vi "Weighted Array Mean & SDV.vi"(4 "Reject NaN, +/-Inf (T)":bool=TRUE, 6 "Reject Negative Weights (F)":bool, 8 "Error In":errorcluster, 9 "Weight Array":dbl[](array[numeric]), 11 "Array":dbl[](array[numeric])) -> (0 "Error Out":errorcluster, 1 "SDV (weighted)":dbl, 2 "SDV (classic)":dbl, 3 "Average Value (weighted)":dbl, 5 "Average Value (classic)":dbl, 7 "Effective # Elements":i32)   [LabVIEW 2021, in "Math.lvlib"]
doc: "Compute a weighted average of the input <B>Array</B> A using the provided <B>Weight Array</B> w:\n\n<A> = (Sum(w_i A_i)_{i = 1....N})/(Sum(w_i)_{i = 1....N})\n\nwhere {A_i}_{i = 1....N} is the input <B>Array</B> and {w_i}_{i = 1....N} is the <B>Weight Array</B>.\n\nIf <B>Reject Negative Weights</B> is true, only the term with w_i >= 0 are retained in both sums.\n\nIf the two arrays have different sizes, the unweighted mean of <B>Array</B> is returned.\n\nTo reject NaN values in the calculation, use the <B>Reject NaN</B> flag."
uses:
  <userlib>/_OpenG.lib/array/array.llb/Filter 1D Array (DBL)__ogtk.vi
  <userlib>/_OpenG.lib/array/array.llb/Delete Elements from 1D Array (DBL)__ogtk.vi
  Math.lvlib
  <vilib>/Analysis/NI_AALBase.lvlib
  <userlib>/_OpenG.lib/array/array.llb/openg_array.lvlib
panel:
  # "see the AlliGator License on the block diagram (Ctrl+E or Window:Show Block Diagram)"
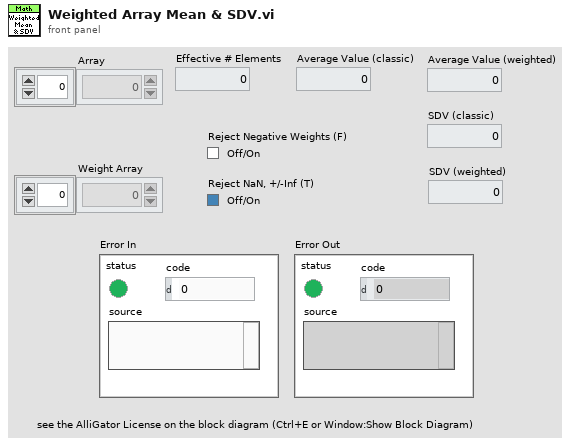
[diagram p1: front panel]
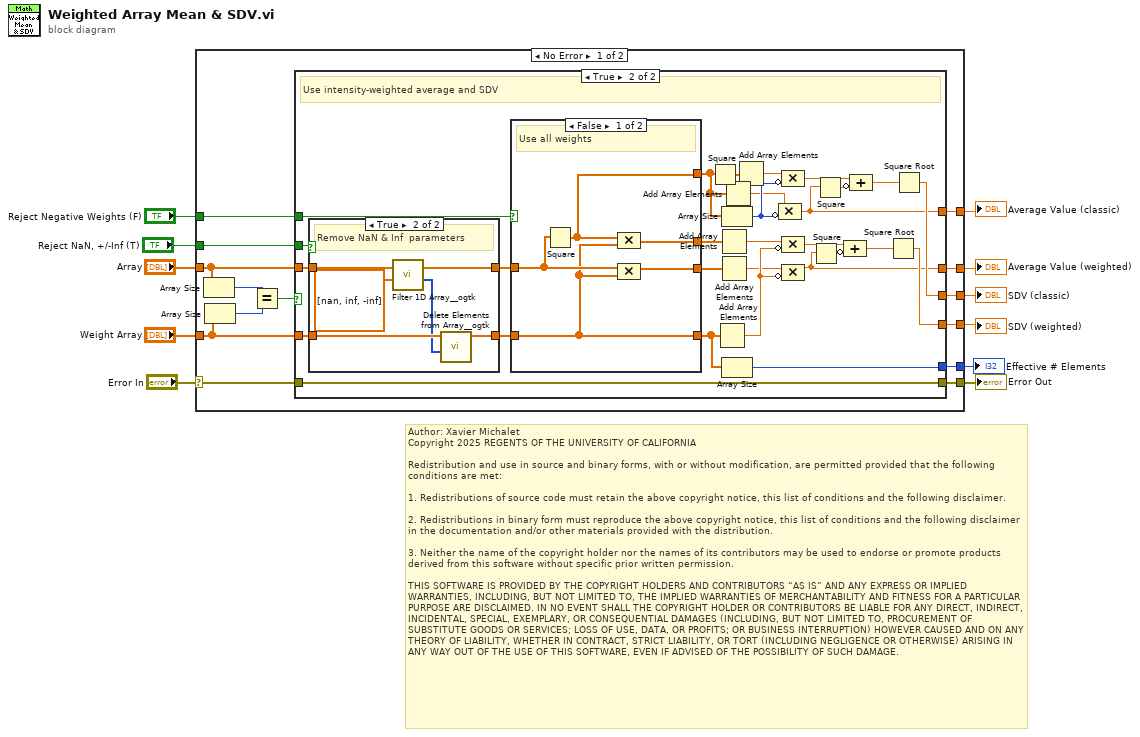
[diagram p0: block diagram]
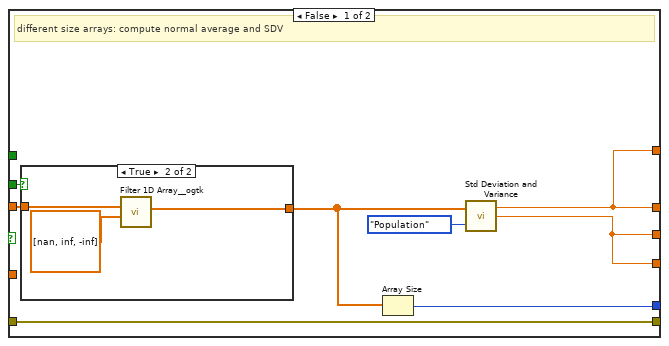
[diagram p2: hidden frame]
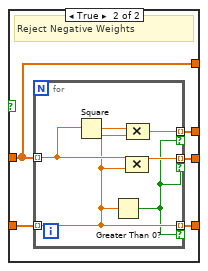
[diagram p5: hidden frame]
diagram:
  # "Author: Xavier Michalet\nCopyright 2025 REGENTS OF THE UNIVERSITY OF CALIFORNIA\n\nRedistribution and use in source and binary forms, with or without modification, are permitted provided that the following conditions are met:\n\n1. Redistributions of source code must retain the above copyright notice, this list of conditions and the following disclaimer.\n\n2. Redistributions in binary form must reproduce the above copyright notice, this list of conditions and the following disclaimer in the documentation and/or other materials provided with the distribution.\n\n3. Neither the name of the copyright holder nor the names of its contributors may be used to endorse or promote products derived from this software without specific prior written permission.\n\nTHIS SOFTWARE IS PROVIDED BY THE COPYRIGHT HOLDERS AND CONTRIBUTORS “AS IS” AND ANY EXPRESS OR IMPLIED WARRANTIES, INCLUDING, BUT NOT LIMITED TO, THE IMPLIED WARRANTIES OF MERCHANTABILITY AND FITNESS FOR A PARTICULAR PURPOSE ARE DISCLAIMED. IN NO EVENT SHALL THE COPYRIGHT HOLDER OR CONTRIBUTORS BE LIABLE FOR ANY DIRECT, INDIRECT, INCIDENTAL, SPECIAL, EXEMPLARY, OR CONSEQUENTIAL DAMAGES (INCLUDING, BUT NOT LIMITED TO, PROCUREMENT OF SUBSTITUTE GOODS OR SERVICES; LOSS OF USE, DATA, OR PROFITS; OR BUSINESS INTERRUPTION) HOWEVER CAUSED AND ON ANY THEORY OF LIABILITY, WHETHER IN CONTRACT, STRICT LIABILITY, OR TORT (INCLUDING NEGLIGENCE OR OTHERWISE) ARISING IN ANY WAY OUT OF THE USE OF THIS SOFTWARE, EVEN IF ADVISED OF THE POSSIBILITY OF SUCH DAMAGE."
  n1 = case shown="No Error" "Error In" {
    selector: "Error In" -> [w17 w91]
    tunnel: "Array" -> [w19 _]
    tunnel: [w23 _] -> w10
    tunnel: [w16 w91] -> w8
    tunnel: "Weight Array" -> [w18 _]
    tunnel: "Reject Negative Weights (F)" -> [w22 _]
    tunnel: "Reject NaN, +/-Inf (T)" -> [w20 _]
    tunnel: [w15 _] -> w4
    tunnel: [w14 _] -> w3
    tunnel: [w13 _] -> w2
    tunnel: [w12 _] -> w1
    frame No Error {
      n2 = Array Size(array=w19) -> (size(s)=w25:i32)
      n3 = Array Size(array=w18) -> (size(s)=w24:i32)
      n4 = Equal?(x=w25, y=w24) -> (x = y?=w21:bool)
      n5 = case shown="True" w21 {
        tunnel: [w28 w45] -> w23
        tunnel: w18 -> [_ w66]
        tunnel: w22 -> [_ w65]
        tunnel: w19 -> [w33 w64]
        tunnel: w20 -> [w32 w60]
        tunnel: w17 -> [w31 w59]
        tunnel: [w31 w59] -> w16
        tunnel: [w30 w55] -> w15
        tunnel: [w30 w47] -> w14
        tunnel: [w28 w40] -> w13
        tunnel: [w26 w38] -> w12
        frame False {
          # "different size arrays: compute normal average and SDV"
          n6 = case shown="True" w32 {
            tunnel: w33 -> [w34 w37]
            tunnel: [w34 w36] -> w27
            frame False {
            }
            frame True {
              n7 = call-poly <userlib>:"Filter 1D Array__ogtk.vi"("items to filter"=dbl[] [nan, inf, -inf] ("Element(s) to Remove"), "array"=w37) -> ("filtered array"=w36:dbl[])  [unwired: 4 in, 1 out]
            }
          }
          n8 = Array Size(array=w27) -> (size(s)=w26:i32)
          n9 = call <vilib>:"Std Deviation and Variance.vi"("X"=w27, "Weighting (Sample)"=enum16{"Sample", "Population"}."Population") -> ("mean"=w28:dbl, "standard deviation"=w30:dbl)  [unwired: 1 out]
        }
        frame True {
          # "Use intensity-weighted average and SDV"
          n10 = case shown="True" w60 {
            tunnel: w66 -> [w67 w74]
            tunnel: w64 -> [w68 w73]
            tunnel: [w68 w72] -> w63
            tunnel: [w67 w70] -> w62
            frame False {
            }
            frame True {
              # "Remove NaN & Inf  parameters"
              n11 = call-poly <userlib>:"Filter 1D Array__ogtk.vi"("items to filter"=dbl[] [nan, inf, -inf] ("Element(s) to Remove"), "array"=w73) -> ("filtered item indices"=w71:i32[], "filtered array"=w72:dbl[])  [unwired: 4 in]
              n12 = call-poly <userlib>:"Delete Elements from Array__ogtk.vi"("indices"=w71, "array"=w74) -> ("array w/ subset deleted"=w70:dbl[])  [unwired: 8 in, 1 out]
            }
          }
          n13 = case shown="False" w65 {
            tunnel: w62 -> [w77 w84]
            tunnel: w63 -> [w78 w80]
            tunnel: [w79 w83] -> w61
            tunnel: [w77 w82] -> w39
            tunnel: [w76 w81] -> w54
            tunnel: [w75 w80] -> w42
            frame False {
              # "Use all weights"
              n14 = Square(x=w78) -> (x^2=w75:dbl[])
              n15 = Compound Arithmetic op=MULTIPLY(w75, w77) -> (w76:dbl[])
              n16 = Compound Arithmetic op=MULTIPLY(w78, w77) -> (w79:dbl[])
            }
            frame True {
              # "Reject Negative Weights"
              n17 = for {
                tunnel: w84 -> [w87] mode=indexing
                tunnel: w80 -> [w89] mode=indexing
                tunnel: [w90] -> w83 mode=indexing if=w85
                tunnel: [w87] -> w82 mode=indexing if=w85
                tunnel: [w86] -> w81 mode=indexing if=w85
                n18 = Square(x=w89) -> (x^2=w88:dbl)
                n19 = Greater Than 0?(x=w87) -> (x > 0?=w85:bool)
                n20 = Compound Arithmetic op=MULTIPLY(w89, w87) -> (w90:dbl)
                n21 = Compound Arithmetic op=MULTIPLY(w88, w87) -> (w86:dbl)
              }
            }
          }
          n22 = Square(x=w42) -> (x^2=w43:dbl[])
          n23 = Add Array Elements(numeric array=w39) -> (sum=w53:dbl)
          n24 = Add Array Elements(numeric array=w54) -> (sum=w49:dbl)
          n25 = Add Array Elements(numeric array=w61) -> (sum=w46:dbl)
          n26 = Array Size(array=w42) -> (size(s)=w50:i32)
          n27 = Array Size(array=w39) -> (size(s)=w38:i32)
          n28 = Add Array Elements(numeric array=w42) -> (sum=w41:dbl)
          n29 = Add Array Elements(numeric array=w43) -> (sum=w57:dbl)
          n30 = Compound Arithmetic op=MULTIPLY(w41, invert w50) -> (w40:dbl)
          n31 = Compound Arithmetic op=MULTIPLY(w57, invert w50) -> (w56:dbl)
          n32 = Compound Arithmetic op=MULTIPLY(w49, invert w53) -> (w52:dbl)
          n33 = Compound Arithmetic op=MULTIPLY(w46, invert w53) -> (w45:dbl)
          n34 = Square(x=w45) -> (x^2=w44:dbl)
          n35 = Square(x=w40) -> (x^2=w51:dbl)
          n36 = Compound Arithmetic op=ADD(w52, invert w44) -> (w48:dbl)
          n37 = Compound Arithmetic op=ADD(w56, invert w51) -> (w58:dbl)
          n38 = Square Root(x=w48) -> (sqrt(x)=w47:dbl)
          n39 = Square Root(x=w58) -> (sqrt(x)=w55:dbl)
        }
      }
    }
    frame Error {
    }
  }
  "Average Value (weighted)" <- w10
  "Error Out" <- w8
  "SDV (classic)" <- w4
  "SDV (weighted)" <- w3
  "Average Value (classic)" <- w2
  "Effective # Elements" <- w1
